vi "mqttCmdCreate.vi"(8 "error in (no error)":errorcluster, 10 "messageID":u16) -> (0 "error out":errorcluster, 3 "mqttCmdPublishReceived out":refnum<class "PublishReceivedMqttMsg.lvclass">)   [LabVIEW 2020, in "PublishReceivedMqttMsg.lvclass"]
uses:
  PublishReceivedMqttMsg.lvclass
  C:/Projects/Libraries/Gore SM 2020/mqtt-LabVIEW/src/class/mqtt/mqttCmd/BaseMqttMsg.lvclass
  mqttTypedef/mqttMessageType.ctl
  mqttTypedef/mqttQOSlevel.ctl
  BaseMqttMsg.lvclass/BaseMqttMsg.ctl
  Properties/Write Datagram.vi
  BaseMqttMsg.lvclass
  mqtt.lvclass
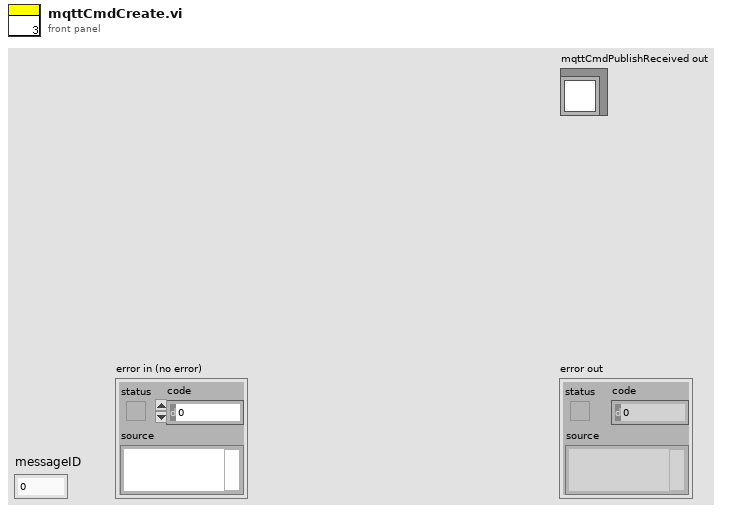
[diagram p1: front panel]
types:
  T1 = typedef "mqtt.lvclass/mqttQOSlevel.ctl" = enum8{"At most once", "At least once", "Exactly once", "Reserved"}
  T2 = typedef "mqtt.lvclass/mqttMessageType.ctl" = enum32{"Reserved", "CONNECT", "CONNACK", "PUBLISH", "PUBACK", "PUBREC", "PUBREL", "PUBCOMP", "SUBSCRIBE", "SUBACK", "UNSUBSCRIBE", "UNSUBACK", "PINGREQ", "PINGRESP", "DISCONNECT", "Reserved2"}
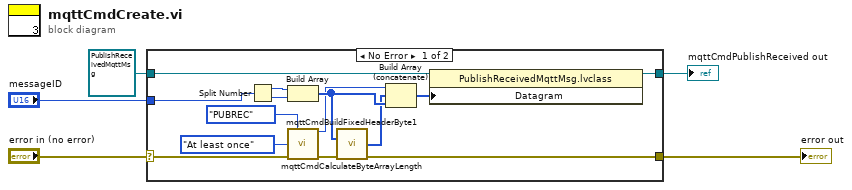
[diagram p0: block diagram]
diagram:
  n1 = case shown="No Error" "error in (no error)" {
    selector: "error in (no error)" -> [w11 w21]
    tunnel: [w7 w21] -> w4
    tunnel: [w10 w20] -> w2
    tunnel: refnum<class "PublishReceivedMqttMsg.lvclass"> refnum ("mqttCmdPublishReceived in") -> [w19 w20]
    tunnel: "messageID" -> [w6 _]
    frame No Error {
      n2 = Split Number(x=w6) -> (hi(x)=w15:u8, lo(x)=w14:u8)
      n3 = Build Array(w15, w14) -> (w16:u8[])
      n4 = call "mqttCmdBuildFixedHeaderByte1.vi"("MessageType"=mqttMessageType."PUBREC", "QoS (At most once)"=mqttQOSlevel."At least once", "error in (no error)"=w11) -> ("byte1"=w12:u8, "error out"=w8:errorcluster)  [unwired: 11 in]
      n5 = call "mqttCmdCalculateByteArrayLength.vi"("byteArry in"=w16, "error in (no error)"=w8) -> ("length out"=w13:u8[], "error out"=w7:errorcluster)  [unwired: 12 in]
      n6 = Build Array (concatenate)(w12, w13, w16) -> (w9:u8[])
      n7 = property class="PublishReceivedMqttMsg.lvclass"(reference=w19, "Datagram"=w9) -> (reference out=w10:refnum<class "PublishReceivedMqttMsg.lvclass">)  [unwired: 1 in, 1 out]
    }
    frame Error {
    }
  }
  "error out" <- w4
  "mqttCmdPublishReceived out" <- w2
